vi "Ref_Mask _ch_11-20.vi"(0 "Mask Ch 11":refnum<vi>, 1 "Mask Ch 12":refnum<vi>, 2 "Mask Ch 13":refnum<vi>, 3 "Mask Ch 14":refnum<vi>, 4 "Mask Ch 15":refnum<vi>, 5 "Mask Ch 16":refnum<vi>, 6 "Mask Ch 17":refnum<vi>, 7 "Mask Ch 18":refnum<vi>, 8 "Mask Ch 19":refnum<vi>, 9 "Mask Ch 20":refnum<vi>, 14 "Init_F":bool=TRUE) -> (18 "Mask Ch 19 out":refnum<vi>, 19 "Mask Ch 20 out":refnum<vi>, 20 "Mask Ch 11 out":refnum<vi>, 21 "Mask Ch 12 out":refnum<vi>, 22 "Mask Ch 13 out":refnum<vi>, 23 "Mask Ch 14 out":refnum<vi>, 24 "Mask Ch 15 out":refnum<vi>, 25 "Mask Ch 16 out":refnum<vi>, 26 "Mask Ch 17 out":refnum<vi>, 27 "Mask Ch 18 out":refnum<vi>)   [LabVIEW 2017]
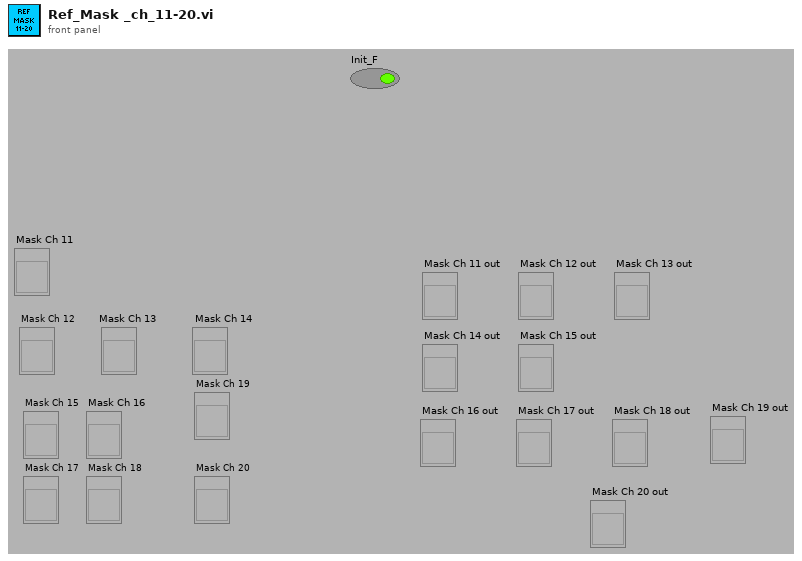
[diagram p1: front panel]
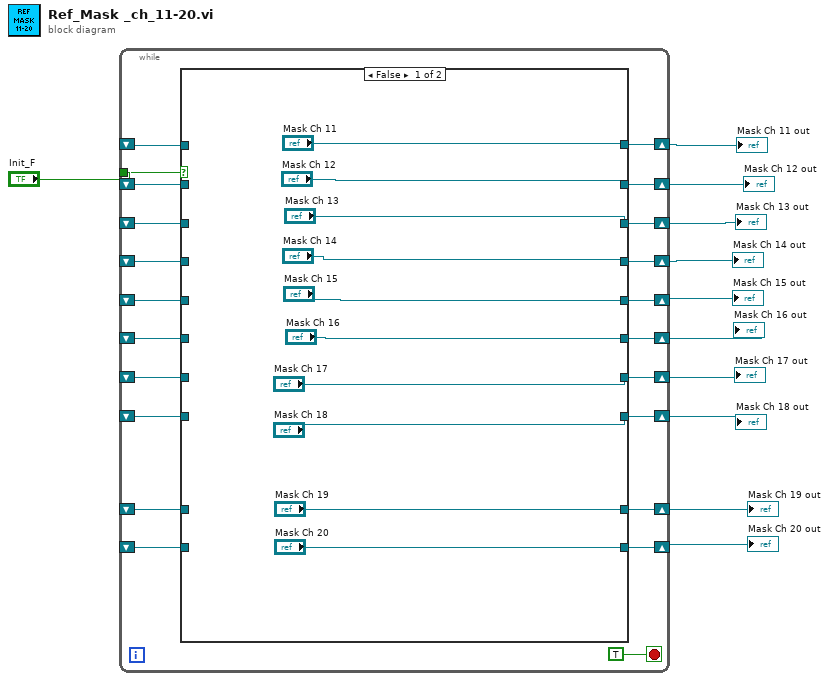
[diagram p0: block diagram]
diagram:
  n1 = while {
    shift-right: [w32] -> w10
    shift-left: _ -> [w31]
    tunnel: "Init_F" -> [w30]
    shift-right: [w29] -> w9
    shift-left: _ -> [w22]
    shift-right: [w28] -> w8
    shift-left: _ -> [w21]
    shift-right: [w27] -> w7
    shift-left: _ -> [w16]
    shift-right: [w26] -> w6
    shift-left: _ -> [w20]
    shift-right: [w25] -> w5
    shift-left: _ -> [w19]
    shift-right: [w24] -> w4
    shift-left: _ -> [w18]
    shift-right: [w23] -> w3
    shift-left: _ -> [w17]
    shift-right: [w15] -> w2
    shift-left: _ -> [w13]
    shift-right: [w14] -> w1
    shift-left: _ -> [w12]
    stop <- TRUE stop-if-true
    n2 = case shown="False" w30 {
      tunnel: ["Mask Ch 11" w53] -> w32
      tunnel: w31 -> [_ w53]
      tunnel: ["Mask Ch 12" w46] -> w29
      tunnel: ["Mask Ch 13" w47] -> w28
      tunnel: ["Mask Ch 14" w48] -> w27
      tunnel: ["Mask Ch 15" w49] -> w26
      tunnel: ["Mask Ch 16" w50] -> w25
      tunnel: ["Mask Ch 17" w51] -> w24
      tunnel: ["Mask Ch 18" w52] -> w23
      tunnel: w22 -> [_ w46]
      tunnel: w21 -> [_ w47]
      tunnel: w20 -> [_ w49]
      tunnel: w19 -> [_ w50]
      tunnel: w18 -> [_ w51]
      tunnel: w17 -> [_ w52]
      tunnel: w16 -> [_ w48]
      tunnel: ["Mask Ch 19" w45] -> w15
      tunnel: ["Mask Ch 20" w44] -> w14
      tunnel: w13 -> [_ w45]
      tunnel: w12 -> [_ w44]
      frame False {
      }
      frame True {
      }
    }
  }
  "Mask Ch 11 out" <- w10
  "Mask Ch 12 out" <- w9
  "Mask Ch 13 out" <- w8
  "Mask Ch 14 out" <- w7
  "Mask Ch 15 out" <- w6
  "Mask Ch 16 out" <- w5
  "Mask Ch 17 out" <- w4
  "Mask Ch 18 out" <- w3
  "Mask Ch 19 out" <- w2
  "Mask Ch 20 out" <- w1
